vi "create basic config file.vi"   [LabVIEW 2018]
uses:
  <vilib>/Utility/config.llb/Write Key (Boolean).vi
  <vilib>/Utility/config.llb/Write Key (String).vi
  <vilib>/Utility/config.llb/Write Key (I32).vi
  <vilib>/Utility/config.llb/Write Key (U32).vi
  <vilib>/Utility/config.llb/NI_LVConfig.lvlib
types:
  T1 = typedef "NI_LVConfig.lvlib/Config Data RefNum.ctl" = refnum<k1>
  T2 = cluster{"Time":bool[], "Tcs":bool[], "RTDs":bool[], "HS VI":bool[], "AI":bool[], "LS VI":bool[], "Torque":bool[], "Pulser":bool[]}
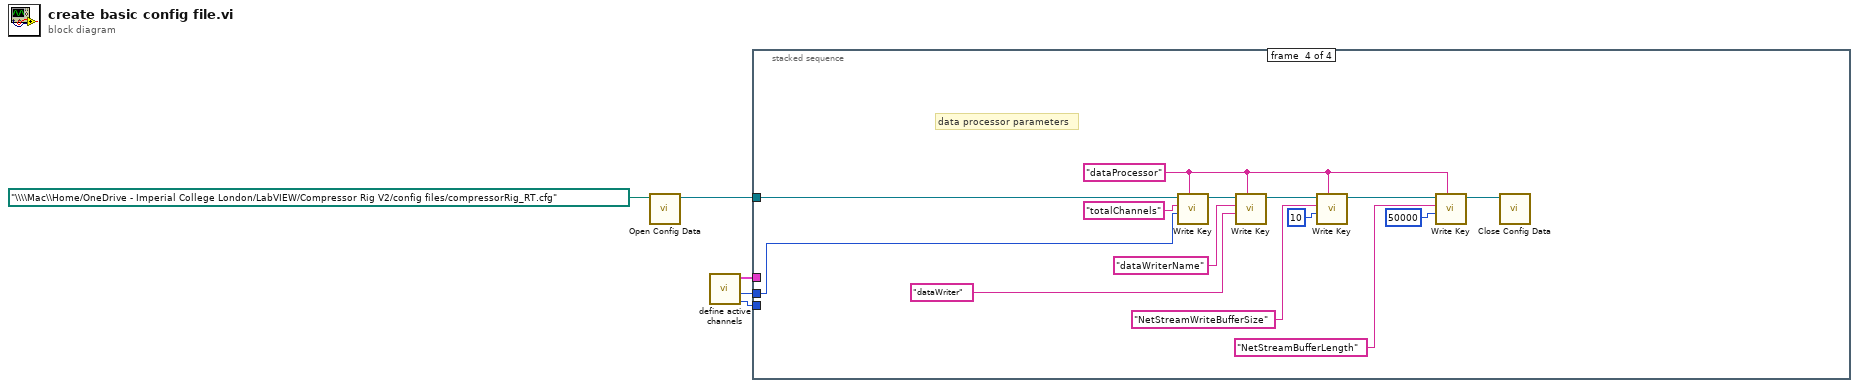
[diagram p0: block diagram]
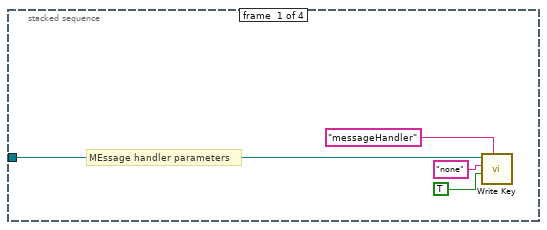
[diagram p2: hidden frame]
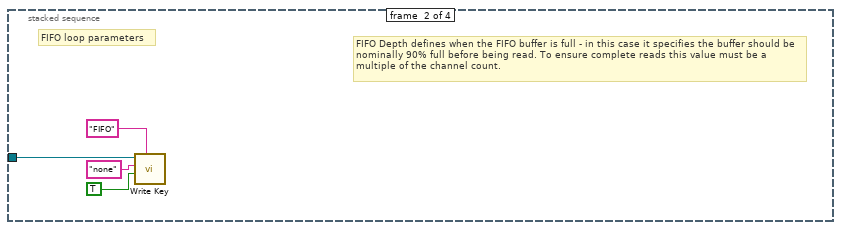
[diagram p3: hidden frame]
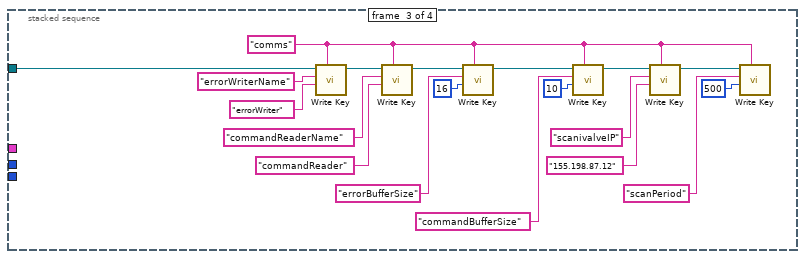
[diagram p4: hidden frame]
diagram:
  n1 = call <vilib>:"Open Config Data.vi"("configuration file path"=path "\\\\Mac\\Home/OneDrive - Imperial College London/LabVIEW/Compressor Rig V2/config files/compressorRig_RT.cfg") -> ("refnum"=w1:T1)  [unwired: 8 in, 2 out]
  n2 = call "define active channels.vi"() -> ("active channels"=w3:i16, "total channel count"=w5:i32, "Active channels"=w4:T2)  [unwired: 9 in]
  n3 = stacked-sequence {
    tunnel: w5 -> [_ _ _ w45]
    tunnel: w4 -> [_ _ _ _]
    tunnel: w3 -> [_ _ _ _]
    tunnel: w1 -> [w6 w10 w31 w46]
    frame #0 {
      # "MEssage handler parameters"
      n4 = call-poly <vilib>:"Write Key.vi"("section"="messageHandler", "value"=TRUE, "key"="none", "refnum"=w6) -> ()  [unwired: 5 in, 3 out]
    }
    frame #1 {
      # "FIFO loop parameters"
      # "FIFO Depth defines when the FIFO buffer is full - in this case it specifies the buffer should be nominally 90% full before being read. To ensure complete reads this value must be a multiple of the channel count."
      n5 = call-poly <vilib>:"Write Key.vi"("section"="FIFO", "value"=TRUE, "key"="none", "refnum"=w10) -> ()  [unwired: 5 in, 3 out]
    }
    frame #2 {
      w20 = "comms" ("section")
      n6 = call-poly <vilib>:"Write Key.vi"("section"=w20, "value"="errorWriter" ("Parameters.error writer name"), "key"="errorWriterName", "refnum"=w31) -> ("refnum out"=w27:T1)  [unwired: 5 in, 2 out]
      n7 = call-poly <vilib>:"Write Key.vi"("section"=w20, "value"="commandReader" ("Parameters.command reader name"), "key"="commandReaderName", "refnum"=w27) -> ("refnum out"=w26:T1)  [unwired: 5 in, 2 out]
      n8 = call-poly <vilib>:"Write Key.vi"("section"=w20, "value"=16 ("Parameters.error buffer size"), "key"="errorBufferSize", "refnum"=w26) -> ("refnum out"=w25:T1)  [unwired: 5 in, 2 out]
      n9 = call-poly <vilib>:"Write Key.vi"("section"=w20, "value"=10 ("Parameters.command buffer size"), "key"="commandBufferSize", "refnum"=w25) -> ("refnum out"=w22:T1)  [unwired: 5 in, 2 out]
      n10 = call-poly <vilib>:"Write Key.vi"("section"=w20, "value"="155.198.87.12" ("Parameters.scanivalveIP"), "key"="scanivalveIP", "refnum"=w22) -> ("refnum out"=w14:T1)  [unwired: 5 in, 2 out]
      n11 = call-poly <vilib>:"Write Key.vi"("section"=w20, "value"=u16 500 ("Parameters.scanivalvePeriod"), "key"="scanPeriod", "refnum"=w14) -> ()  [unwired: 5 in, 3 out]
    }
    frame #3 {
      w40 = "dataProcessor" ("Parameters.Data stream.data writer name")
      # "data processor parameters"
      n12 = call-poly <vilib>:"Write Key.vi"("section"=w40, "value"=w45, "key"="totalChannels" ("Parameters.Data stream.data writer name"), "refnum"=w46) -> ("refnum out"=w44:T1)  [unwired: 5 in, 2 out]
      n13 = call-poly <vilib>:"Write Key.vi"("section"=w40, "value"="dataWriter" ("Parameters.Data stream.data writer name"), "key"="dataWriterName" ("Parameters.Data stream.data writer name"), "refnum"=w44) -> ("refnum out"=w35:T1)  [unwired: 5 in, 2 out]
      n14 = call-poly <vilib>:"Write Key.vi"("section"=w40, "value"=10 ("Parameters.Data stream.data buffer size"), "key"="NetStreamWriteBufferSize" ("Parameters.Data stream.data writer name"), "refnum"=w35) -> ("refnum out"=w34:T1)  [unwired: 5 in, 2 out]
      n15 = call-poly <vilib>:"Write Key.vi"("section"=w40, "value"=u32 50000 ("Parameters.data stream.NS Buffer length"), "key"="NetStreamBufferLength" ("Parameters.Data stream.data writer name"), "refnum"=w34) -> ("refnum out"=w33:T1)  [unwired: 5 in, 2 out]
      n16 = call <vilib>:"Close Config Data.vi"("refnum"=w33) -> ()  [unwired: 9 in, 2 out]
    }
  }
